vi "mergeDotNetInvokeNode.vi"   [LabVIEW 2020]
doc: "Invokes a method or action on a reference. Most methods have associated parameters."
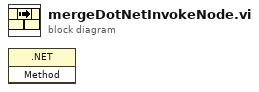
[diagram p0: block diagram]
diagram:
  n1 = invoke class=".NET" method=#-1() -> ()  [unwired: 3 in, 3 out]
